vi "自检dll.vi"() -> ()   [LabVIEW 2016]
panel:
  out "file or folder exists?":bool caption="文件或文件夹存在？"
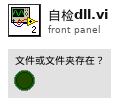
[diagram p1: front panel]
types:
  T1 = enum32{"Invalid", "Standard", "Closed", "Hidden", "Minimized", "Maximized"}
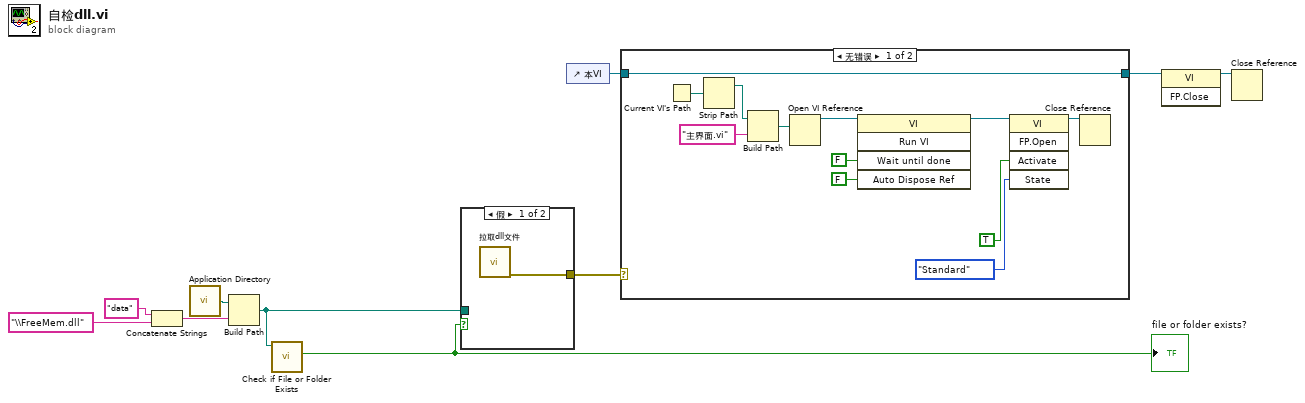
[diagram p0: block diagram]
diagram:
  n1 = Concatenate Strings("data" ("名称或相对路径"), "\\FreeMem.dll" ("名称或相对路径")) -> (w9:string)
  n2 = call <vilib>:"Application Directory.vi"() -> ("Application Directory"=w7:path)
  n3 = Build Path(base path=w7, name or relative path=w9) -> (appended path=w5:path)
  n4 = call <vilib>:"Check if File or Folder Exists.vi"("path"=w5) -> ("file or folder exists?"=w6:bool)  [unwired: 8 in, 2 out]
  "file or folder exists?" <- w6
  n5 = case shown="假" w6 {
    tunnel: w5 -> [_ _]
    tunnel: [w11 _] -> w4
    frame False {
      n6 = call "拉取dll文件.vi"() -> ("error out"=w11:errorcluster)  [unwired: 11 in]
    }
    frame True {
    }
  }
  n7 = control-ref of="本VI"() -> (w1:refnum<vi>)
  n8 = case shown="无错误" w4 {
    tunnel: [w12 w24] -> w3
    tunnel: w1 -> [w12 w24]
    frame No Error {
      n9 = Current VI's Path() -> (path=w13:path)
      n10 = Strip Path(path=w13) -> (stripped path=w14:path)  [unwired: 1 out]
      n11 = Build Path(base path=w14, name or relative path="主界面.vi" ("名称或相对路径")) -> (appended path=w16:path)
      n12 = Open VI Reference(vi path=w16) -> (vi reference=w17:refnum<vi>)  [unwired: 5 in, 1 out]
      n13 = invoke class="VI" method="Run VI"(reference=w17, "Wait until done"=FALSE ("结束前等待"), "Auto Dispose Ref"=FALSE ("自动销毁引用")) -> (reference out=w20:refnum<vi>)  [unwired: 2 in, 4 out]
      n14 = invoke class="VI" method="FP.Open"(reference=w20, "Activate"=TRUE ("激活？"), "State"=T1."Standard" ("状态")) -> (reference out=w23:refnum<vi>)  [unwired: 2 in, 4 out]
      n15 = Close Reference(reference=w23) -> ()  [unwired: 1 in, 1 out]
    }
    frame Error {
    }
  }
  n16 = invoke class="VI" method="FP.Close"(reference=w3) -> (reference out=w2:refnum<vi>)  [unwired: 2 in, 2 out]
  n17 = Close Reference(reference=w2) -> ()  [unwired: 1 in, 1 out]
